vi "Write parity.vi"(8 "error in (no error)":errorcluster, 10 "parity":enum16{"None", "Odd", "Even", "Mark", "Space"}(ring), 11 "Serial Data Unit in":refnum<class "Serial Data Unit.lvclass">) -> (0 "error out":errorcluster, 3 "Serial Data Unit out":refnum<class "Serial Data Unit.lvclass">)   [LabVIEW 2021, in "Serial Data Unit.lvclass"]
uses:
  Serial Data Unit.lvclass
  Serial Data Unit.lvclass/Serial Data Unit.ctl
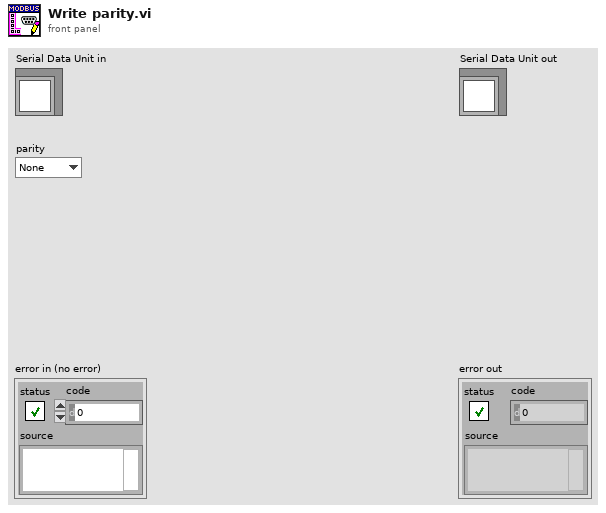
[diagram p1: front panel]
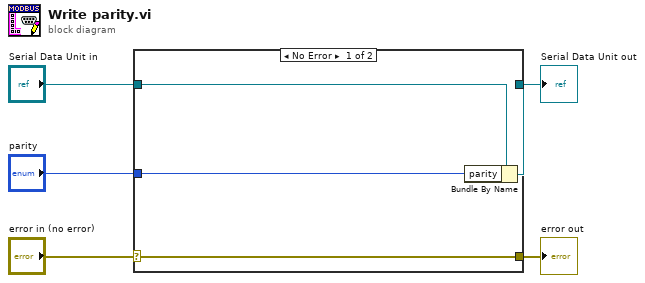
[diagram p0: block diagram]
diagram:
  n1 = case shown="No Error" "error in (no error)" {
    selector: "error in (no error)" -> [w9 w10]
    tunnel: [w9 w10] -> w4
    tunnel: [w7 w11] -> w2
    tunnel: "Serial Data Unit in" -> [w8 w11]
    tunnel: "parity" -> [w6 _]
    frame No Error {
      n2 = Bundle By Name(cluster=w8, "parity"=w6) -> (w7:refnum<class "Serial Data Unit.lvclass">)
    }
    frame Error {
    }
  }
  "error out" <- w4
  "Serial Data Unit out" <- w2
